vi "Plot_Server_Data.vi"() -> ()   [LabVIEW 2015]
uses:
  Anemometry/Anemometry Sub Vis/Controls/Server_Comms.ctl
  Anemometry/Anemometry Sub Vis/File/Setup_Filetype.ctl
  Anemometry/Anemometry Sub Vis/Globals/Preference_global.vi
panel:
  out "LastUpdated":string="Tue, May 12, 2015 at 11:28"
  in  "Throwback\n(mins)":dbl format="%.1f"
  in  "Precision":i32=2
  in  "Save 3":bool
  out "Plot 3 Chs":string[](array[string])
  in  "Save 2":bool
  out "Plot 2 Chs":string[](array[string])
  in  "Save 1":bool
  out "Plot 1 Chs":string[](array[string])
  in  "Save plot number":T1(ring)
  in  "Selector 1":i32[](listbox)
  in  "Search 1":string="Null" caption="Search:"
  in  "Search 2":string="Null" caption="Search:"
  in  "Search 3":string="Null" caption="Search:"
  out "Plot 3":cluster{"Times":dbl[], "Output array":dbl[]}[](graph)
  in  "Selector 3":i32[](listbox)
  out "Plot 2":cluster{"Times":dbl[], "Output array":dbl[]}[](graph)
  in  "Selector 2":i32[](listbox)
  in  "stop":bool=TRUE
  in  "Mode":T2(ring)=enum."Display data over specified period:"
  out "Plot 1":cluster{"Times":dbl[], "Output array":dbl[]}[](graph)
  in  "History\n(mins)":dbl=20.0 format="%.1f"
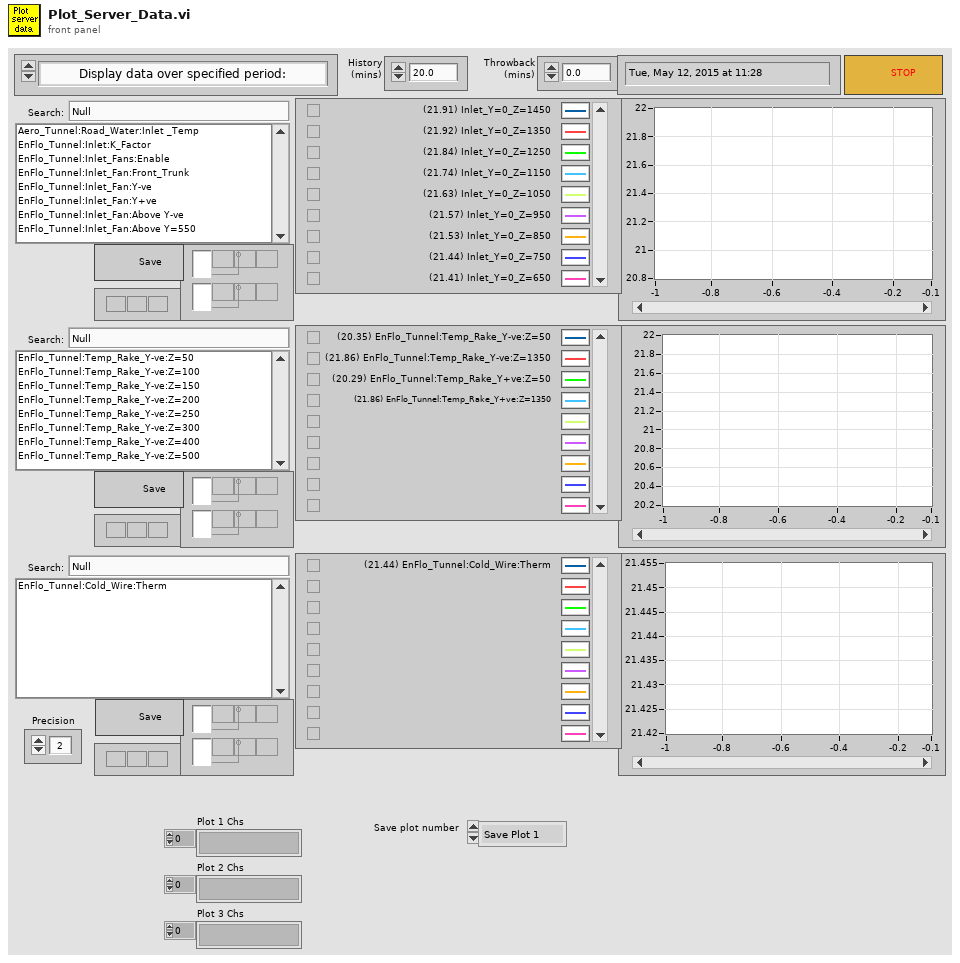
[diagram p1: front panel]
types:
  T1 = enum16{"Save Plot 1", "Save Plot 2", "Save Plot 3"}
  T2 = enum16{"Display full time history", "Display data over specified period:"}
  T3 = typedef "Server_Comms.ctl" = enum16{"Server Link Healthy", "Do Not Link To Server"}
  T4 = typedef "Setup_Filetype.ctl" = enum16{"Measurement Setups", "Calibration Setups", "General", "Results File Plotter Setups", "Speed Calib Tweaks"}
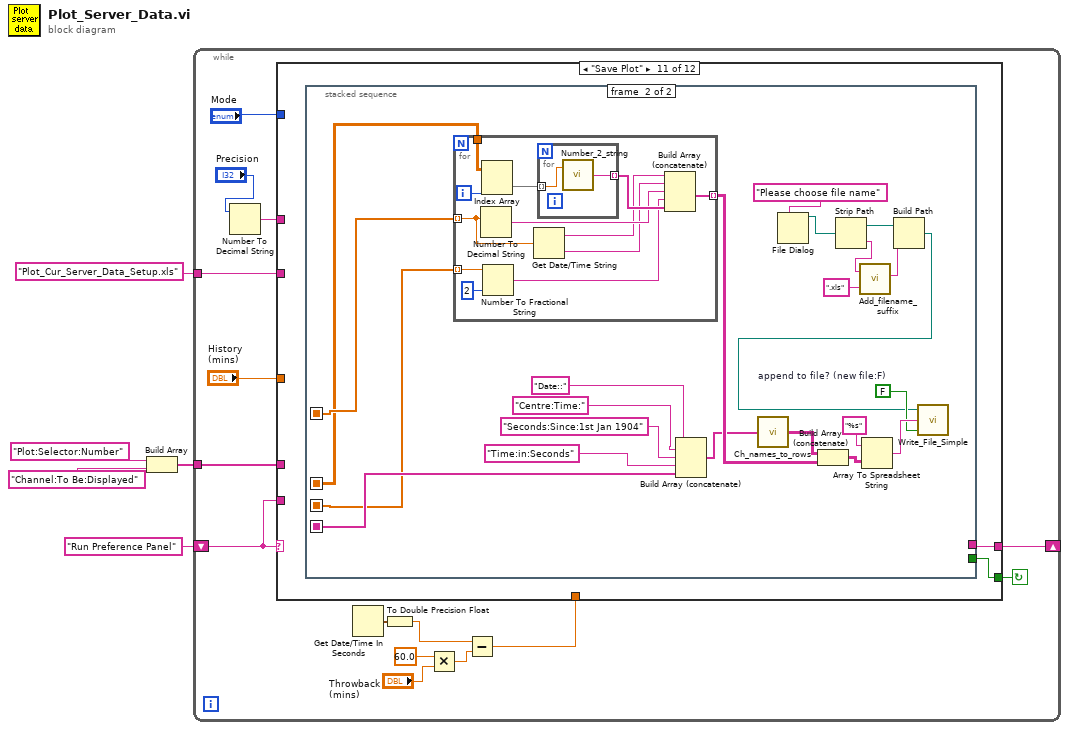
[diagram p0: block diagram]
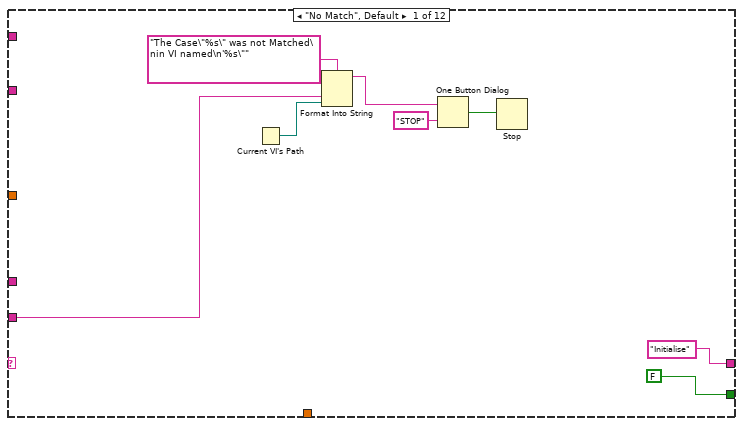
[diagram p2: hidden frame]
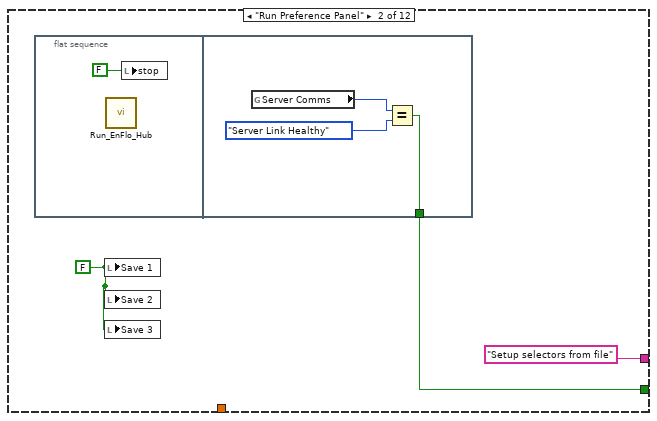
[diagram p3: hidden frame]
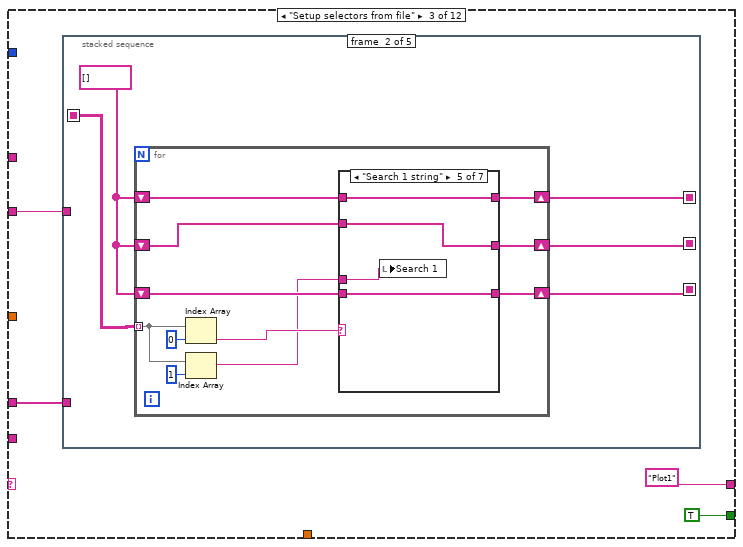
[diagram p4: hidden frame]
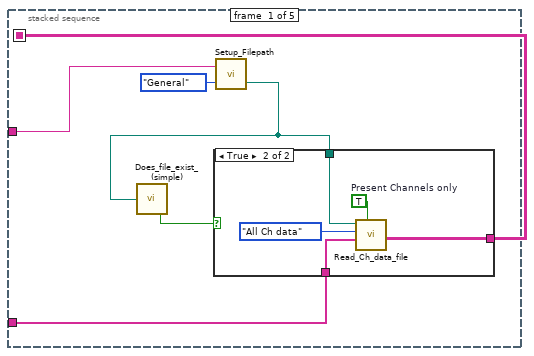
[diagram p5: hidden frame]
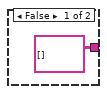
[diagram p6: hidden frame]
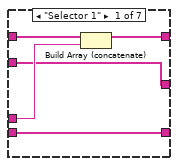
[diagram p7: hidden frame]
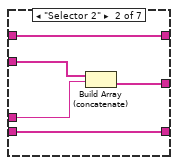
[diagram p8: hidden frame]
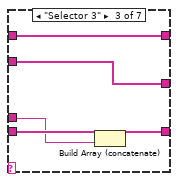
[diagram p9: hidden frame]
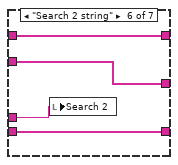
[diagram p11: hidden frame]
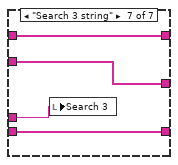
[diagram p12: hidden frame]
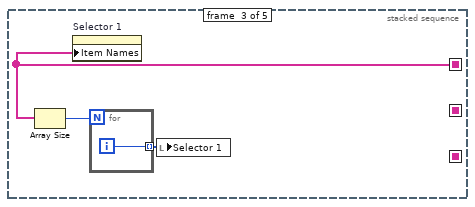
[diagram p13: hidden frame]
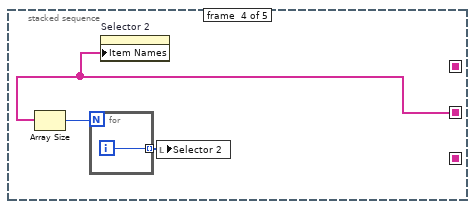
[diagram p14: hidden frame]
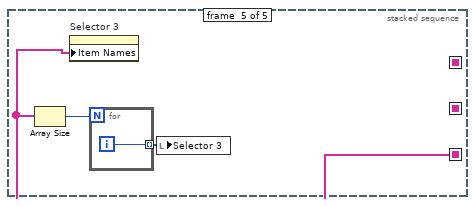
[diagram p15: hidden frame]
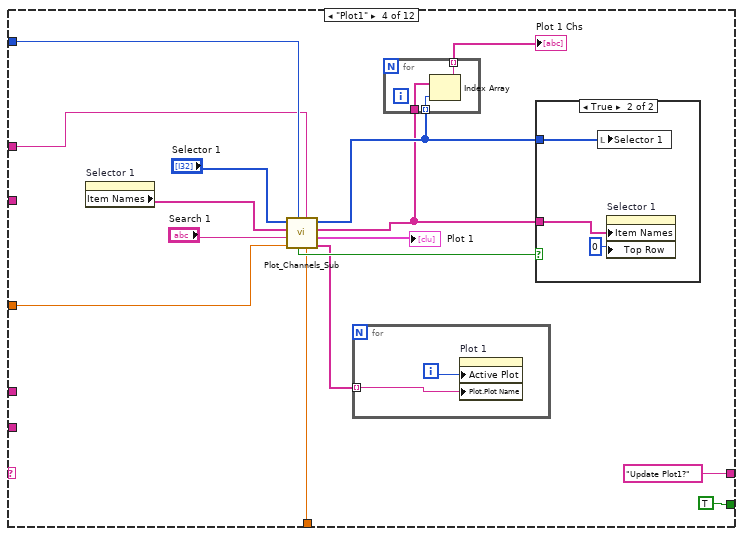
[diagram p16: hidden frame]
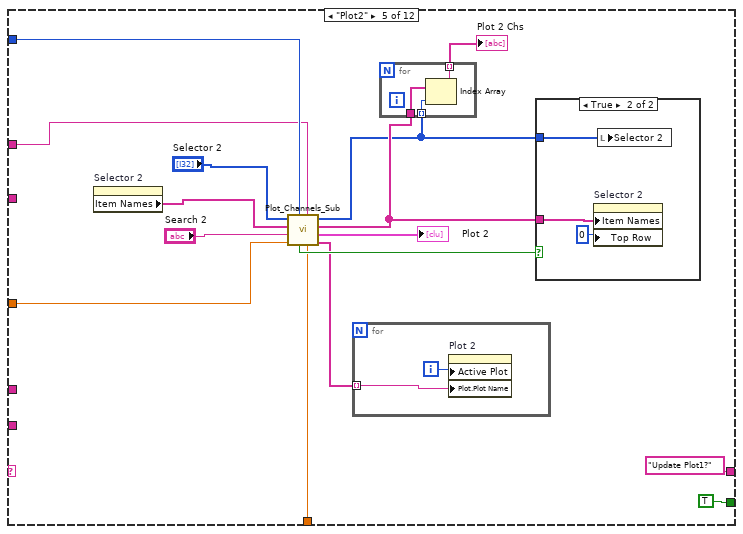
[diagram p18: hidden frame]
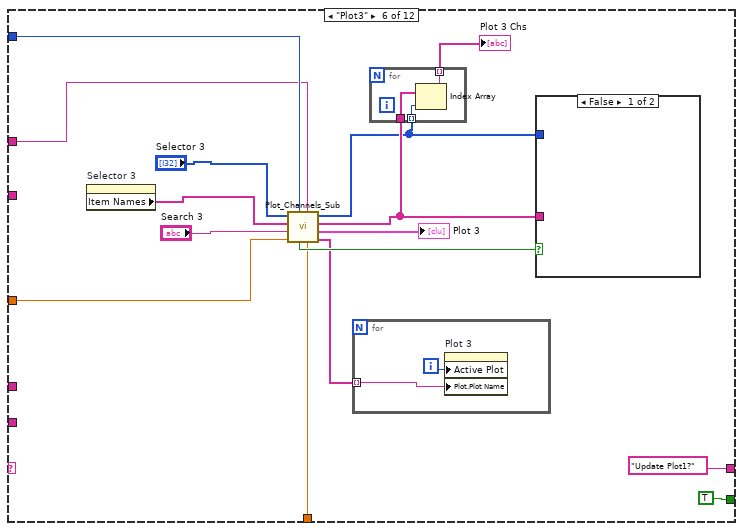
[diagram p20: hidden frame]
diagram:
  n1 = Build Array("Plot:Selector:Number", "Channel:To Be:Displayed") -> (w2:string[])
  n2 = while {
    shift-left: "Run Preference Panel" -> [w18]
    shift-right: [w19] -> _
    tunnel: w2 -> [w15]
    tunnel: "Plot_Cur_Server_Data_Setup.xls" -> [w14]
    stop <- w20 continue-if-true
    n3 = Number To Decimal String(number="Precision") -> (decimal integer string=w12:string)  [unwired: 1 out]
    n4 = Get Date/Time In Seconds() -> (seconds since 1Jan1904=w11:timestamp)
    n5 = To Double Precision Float(number=w11) -> (double precision float=w7:dbl)
    n6 = Multiply(x=60.0, y="Throwback\n(mins)") -> (x*y=w8:dbl)
    n7 = Subtract(x=w7, y=w8) -> (x-y=w6:dbl)
    n8 = case shown="\"Save Plot\"" w18 {
      tunnel: [FALSE w30 TRUE TRUE TRUE TRUE TRUE TRUE TRUE TRUE w305 w370] -> w20
      tunnel: ["Initialise" "Setup selectors from file" "Plot1" "Update Plot1?" "Update Plot1?" "Update Plot1?" w180 w201 w221 w253 w306 "Update Plot1?" ("t")] -> w19
      tunnel: w18 -> [w23 _ _ _ _ _ _ _ _ _ _ _]
      tunnel: "Mode" -> [_ _ _ w117 w144 w167 _ _ _ _ _ _]
      tunnel: "History\n(mins)" -> [_ _ _ w116 w143 w166 _ _ _ _ _ _]
      tunnel: w15 -> [_ _ w36 _ _ _ _ _ _ _ _ w374]
      tunnel: w14 -> [_ _ w37 _ _ _ _ _ _ _ _ w373]
      tunnel: w12 -> [_ _ _ w111 w134 w157 _ _ _ _ _ _]
      tunnel: w6 -> [_ _ _ w110 w133 w156 _ _ _ _ _ _]
      frame "No Match", Default {
        n9 = Current VI's Path() -> (path=w22:path)
        n10 = Format Into String(format string="The Case\"%s\" was not Matched\nin VI named\n'%s\"" ("Format String"), w23, w22) -> (resulting string=w26:string)  [unwired: 2 in, 1 out]
        n11 = One Button Dialog(message=w26, button name ("OK")="STOP") -> (true=w24:bool)
        n12 = Stop(stop? (T)=w24) -> ()
      }
      frame "Run Preference Panel" {
        w29 = FALSE ("Save 1")
        n13 = flat-sequence {
          tunnel: [w33] -> w30
          frame #0 {
            n14 = call "Run_EnFlo_Hub.vi"() -> ()  [unwired: 8 out]
            n15 = local write "stop"(FALSE ("stop")) -> ()
          }
          frame #1 {
            n16 = global read "Preference_global.vi" "Server Comms"() -> (w34:T3)
            n17 = Equal?(x=w34, y=Server_Comms."Server Link Healthy" ("Server Comms")) -> (x = y?=w33:bool)
          }
        }
        n18 = local write "Save 1"(w29) -> ()
        n19 = local write "Save 2"(w29) -> ()
        n20 = local write "Save 3"(w29) -> ()
      }
      frame "Setup selectors from file" {
        n21 = stacked-sequence {
          seq-local: [w43 _ _ _ _] -> [_ w56 _ _ _]
          seq-local: [_ w54 _ _ _] -> [_ _ w100 _ _]
          seq-local: [_ w52 _ _ _] -> [_ _ _ w102 _]
          seq-local: [_ w53 _ _ _] -> [_ _ _ _ w106]
          tunnel: w37 -> [w42 _ _ _ _]
          tunnel: w36 -> [w44 _ _ _ _]
          frame #0 {
            n22 = call "Setup_Filepath.vi"("Setup File Type"=Setup_Filetype."General", "Filename in"=w42) -> ("Filename Out"=w41:path)  [unwired: 1 out]
            n23 = call "Does_file_exist_(simple).vi"("Pathname"=w41) -> ("exists?"=w45:bool)
            n24 = case shown="True" w45 {
              tunnel: w41 -> [_ w51]
              tunnel: w44 -> [_ w50]
              tunnel: [string[][] [] ("Channel Values") w47] -> w43
              frame False {
              }
              frame True {
                w49 = TRUE  # Present Channels only
                n25 = call "Read_Ch_data_file.vi"("Present Channels only"=w49, "Present Channels"=w50, "Output"=enum16{"All Ch data", "The last few rows"}."All Ch data", "Filename"=w51) -> ("Channel Values"=w47:string[][])  [unwired: 1 in, 4 out]
              }
            }
          }
          frame #1 {
            w55 = string[] []
            n26 = for {
              shift-right: [w62] -> w54
              shift-left: w55 -> [w63]
              tunnel: w56 -> [w64] mode=indexing
              shift-right: [w60] -> w52
              shift-left: w55 -> [w61]
              shift-right: [w58] -> w53
              shift-left: w55 -> [w59]
              n27 = Index Array(array=w64, index=0 ("Index")) -> (element=w66:string)
              n28 = Index Array(array=w64, index=1 ("Index")) -> (element=w57:string)
              n29 = case shown="\"Search 1 string\"" w66 {
                tunnel: w63 -> [w72 w77 w78 w84 w88 w92 w96]
                tunnel: [w71 w77 w78 w84 w88 w92 w96] -> w62
                tunnel: w57 -> [w70 w74 w80 _ w86 w90 w94]
                tunnel: w61 -> [w69 w75 w79 w85 w89 w93 w97]
                tunnel: [w69 w73 w79 w85 w89 w93 w97] -> w60
                tunnel: w59 -> [w68 w76 w82 w83 w87 w91 w95]
                tunnel: [w68 w76 w81 w83 w87 w91 w95] -> w58
                frame "Selector 1" {
                  n30 = Build Array (concatenate)(w72, w70) -> (w71:string[])
                }
                frame "Selector 2" {
                  n31 = Build Array (concatenate)(w75, w74) -> (w73:string[])
                }
                frame "Selector 3" {
                  n32 = Build Array (concatenate)(w82, w80) -> (w81:string[])
                }
                frame "No Match", Default {
                }
                frame "Search 1 string" {
                  n33 = local write "Search 1"(w86) -> ()
                }
                frame "Search 2 string" {
                  n34 = local write "Search 2"(w90) -> ()
                }
                frame "Search 3 string" {
                  n35 = local write "Search 3"(w94) -> ()
                }
              }
            }
          }
          frame #2 {
            n36 = Array Size(array=w100) -> (size(s)=w99:i32)
            n37 = property on="Selector 1" class="LstBox (strict)"("Item Names"=w100) -> ()  [unwired: 2 in, 2 out]
            n38 = for {
              N: w99 -> [_]
              tunnel: [w101] -> w98 mode=indexing
              i -> [w101]
            }
            n39 = local write "Selector 1"(w98) -> ()
          }
          frame #3 {
            n40 = Array Size(array=w102) -> (size(s)=w104:i32)
            n41 = for {
              N: w104 -> [_]
              tunnel: [w105] -> w103 mode=indexing
              i -> [w105]
            }
            n42 = property on="Selector 2" class="LstBox (strict)"("Item Names"=w102) -> ()  [unwired: 2 in, 2 out]
            n43 = local write "Selector 2"(w103) -> ()
          }
          frame #4 {
            n44 = Array Size(array=w106) -> (size(s)=w108:i32)
            n45 = property on="Selector 3" class="LstBox (strict)"("Item Names"=w106) -> ()  [unwired: 2 in, 2 out]
            n46 = for {
              N: w108 -> [_]
              tunnel: [w109] -> w107 mode=indexing
              i -> [w109]
            }
            n47 = local write "Selector 3"(w107) -> ()
          }
        }
      }
      frame "Plot1" {
        n48 = property on="Selector 1" class="LstBox (strict)"() -> ("Item Names"=w119:string[])  [unwired: 2 in, 2 out]
        n49 = call "Plot_Channels_Sub.vi"("End Time"=w110, "precision"=w111, "Mode"=w117, "History (min)"=w116, "Search String"="Search 1", "Selector List In"=w119, "Selector array In"="Selector 1") -> ("Plot Legend"=w115:string[], "Plot"=→"Plot 1":cluster{"Times":dbl[], "Output array":dbl[]}[], "Selector List Out"=w113:string[], "Selector array Out"=w114:i32[], "Selector Changed?"=w121:bool)
        n50 = for {
          tunnel: w115 -> [w128] mode=indexing
          i -> [w129]
          n51 = property on="Plot 1" class="XYGraph (strict)"("Active Plot"=w129, "Plot.Plot Name"=w128) -> ()  [unwired: 2 in, 2 out]
        }
        n52 = for {
          tunnel: w114 -> [w127] mode=indexing
          tunnel: w113 -> [w126]
          tunnel: [w125] -> w112 mode=indexing
          n53 = Index Array(array=w126, index=w127) -> (element=w125:string)
        }
        "Plot 1 Chs" <- w112
        n54 = case shown="True" w121 {
          tunnel: w113 -> [_ w132]
          tunnel: w114 -> [_ w131]
          frame False {
          }
          frame True {
            n55 = local write "Selector 1"(w131) -> ()
            n56 = property on="Selector 1" class="LstBox (strict)"("Item Names"=w132, "Top Row"=0) -> ()  [unwired: 2 in, 2 out]
          }
        }
      }
      frame "Plot2" {
        n57 = property on="Selector 2" class="LstBox (strict)"() -> ("Item Names"=w139:string[])  [unwired: 2 in, 2 out]
        n58 = call "Plot_Channels_Sub.vi"("End Time"=w133, "precision"=w134, "Mode"=w144, "History (min)"=w143, "Search String"="Search 2", "Selector List In"=w139, "Selector array In"="Selector 2") -> ("Plot Legend"=w138:string[], "Plot"=→"Plot 2":cluster{"Times":dbl[], "Output array":dbl[]}[], "Selector List Out"=w137:string[], "Selector array Out"=w136:i32[], "Selector Changed?"=w145:bool)
        n59 = for {
          tunnel: w138 -> [w151] mode=indexing
          i -> [w152]
          n60 = property on="Plot 2" class="XYGraph (strict)"("Active Plot"=w152, "Plot.Plot Name"=w151) -> ()  [unwired: 2 in, 2 out]
        }
        n61 = for {
          tunnel: w136 -> [w150] mode=indexing
          tunnel: w137 -> [w149]
          tunnel: [w148] -> w135 mode=indexing
          n62 = Index Array(array=w149, index=w150) -> (element=w148:string)
        }
        "Plot 2 Chs" <- w135
        n63 = case shown="True" w145 {
          tunnel: w137 -> [_ w154]
          tunnel: w136 -> [_ w155]
          frame False {
          }
          frame True {
            n64 = property on="Selector 2" class="LstBox (strict)"("Item Names"=w154, "Top Row"=0) -> ()  [unwired: 2 in, 2 out]
            n65 = local write "Selector 2"(w155) -> ()
          }
        }
      }
      frame "Plot3" {
        n66 = property on="Selector 3" class="LstBox (strict)"() -> ("Item Names"=w162:string[])  [unwired: 2 in, 2 out]
        n67 = call "Plot_Channels_Sub.vi"("End Time"=w156, "precision"=w157, "Mode"=w167, "History (min)"=w166, "Search String"="Search 3", "Selector List In"=w162, "Selector array In"="Selector 3") -> ("Plot Legend"=w161:string[], "Plot"=→"Plot 3":cluster{"Times":dbl[], "Output array":dbl[]}[], "Selector List Out"=w160:string[], "Selector array Out"=w159:i32[], "Selector Changed?"=w168:bool)
        n68 = for {
          tunnel: w161 -> [w174] mode=indexing
          i -> [w175]
          n69 = property on="Plot 3" class="XYGraph (strict)"("Active Plot"=w175, "Plot.Plot Name"=w174) -> ()  [unwired: 2 in, 2 out]
        }
        n70 = for {
          tunnel: w159 -> [w173] mode=indexing
          tunnel: w160 -> [w172]
          tunnel: [w171] -> w158 mode=indexing
          n71 = Index Array(array=w172, index=w173) -> (element=w171:string)
        }
        "Plot 3 Chs" <- w158
        n72 = case shown="False" w168 {
          tunnel: w160 -> [_ w177]
          tunnel: w159 -> [_ w178]
          frame False {
          }
          frame True {
            n73 = local write "Selector 3"(w178) -> ()
            n74 = property on="Selector 3" class="LstBox (strict)"("Item Names"=w177, "Top Row"=0) -> ()  [unwired: 2 in, 2 out]
          }
        }
      }
      frame "Update Plot1?" {
        n75 = while {
          shift-right: [w198] -> w187
          shift-left: _ -> [w195]
          shift-right: [w197] -> w189
          shift-left: _ -> [w196]
          tunnel: [w196] -> w188
          tunnel: [w195] -> w186
          stop <- FALSE continue-if-true
          n76 = local read "Selector 1"() -> (w198:i32[])
          n77 = local read "Search 1"() -> (w197:string)
        }
        n78 = case shown="False" "Save 1" {
          tunnel: ["Update Plot2?" "Save Plot" ("t")] -> w179
          frame False {
          }
          frame True {
            n79 = local write "Save plot number"(T1."Save Plot 1" ("Save plot number")) -> ()
          }
        }
        n80 = Equal?(x=w187, y=w186) -> (x = y?=w184:bool)
        n81 = Equal?(x=w188, y=w189) -> (x = y?=w185:bool)
        n82 = And(x=w184, y=w185) -> (x .and. y?=w183:bool)
        n83 = Select(t=w179, s=w183, f="Plot1") -> (s? t:f=w180:string)
      }
      frame "Update Plot2?" {
        n84 = while {
          shift-right: [w218] -> w207
          shift-left: _ -> [w215]
          shift-right: [w217] -> w209
          shift-left: _ -> [w216]
          tunnel: [w216] -> w208
          tunnel: [w215] -> w206
          stop <- FALSE continue-if-true
          n85 = local read "Selector 2"() -> (w218:i32[])
          n86 = local read "Search 2"() -> (w217:string)
        }
        n87 = case shown="False" "Save 2" {
          tunnel: ["Update Plot3?" "Save Plot" ("t")] -> w199
          frame False {
          }
          frame True {
            n88 = local write "Save plot number"(T1."Save Plot 2" ("Save plot number")) -> ()
          }
        }
        n89 = Equal?(x=w207, y=w206) -> (x = y?=w204:bool)
        n90 = Equal?(x=w208, y=w209) -> (x = y?=w205:bool)
        n91 = And(x=w204, y=w205) -> (x .and. y?=w203:bool)
        n92 = Select(t=w199, s=w203, f="Plot2") -> (s? t:f=w201:string)
      }
      frame "Update Plot3?" {
        n93 = while {
          shift-right: [w238] -> w227
          shift-left: _ -> [w235]
          shift-right: [w237] -> w229
          shift-left: _ -> [w236]
          tunnel: [w236] -> w228
          tunnel: [w235] -> w226
          stop <- FALSE continue-if-true
          n94 = local read "Selector 3"() -> (w238:i32[])
          n95 = local read "Search 3"() -> (w237:string)
        }
        n96 = case shown="False" "Save 3" {
          tunnel: ["What to do next?" "Save Plot" ("t")] -> w219
          frame False {
          }
          frame True {
            n97 = local write "Save plot number"(T1."Save Plot 3" ("Save plot number")) -> ()
          }
        }
        n98 = Equal?(x=w227, y=w226) -> (x = y?=w224:bool)
        n99 = Equal?(x=w228, y=w229) -> (x = y?=w225:bool)
        n100 = And(x=w224, y=w225) -> (x .and. y?=w223:bool)
        n101 = Select(t=w219, s=w223, f="Plot3") -> (s? t:f=w221:string)
      }
      frame "What to do next?" {
        n102 = Wait (ms)(milliseconds to wait=u32 300) -> ()  [unwired: 1 out]
        n103 = while {
          shift-right: [w269] -> _
          shift-left: _ -> [w268]
          shift-right: [w267] -> _
          shift-left: _ -> [w266]
          shift-right: [w259] -> _
          shift-left: _ -> [w258]
          tunnel: [w261] -> w252
          shift-right: [w255] -> w241
          shift-left: _ -> [w256]
          stop <- FALSE continue-if-true
          n104 = local read "History\n(mins)"() -> (w269:dbl)
          n105 = local read "Mode"() -> (w267:T2)
          n106 = Equal?(x=w269, y=w268) -> (x = y?=w265:bool)
          n107 = Equal?(x=w266, y=w267) -> (x = y?=w264:bool)
          n108 = And(x=w265, y=w264) -> (x .and. y?=w263:bool)
          n109 = Select(t=w258, s=w263, f=0) -> (s? t:f=w260:i32)
          n110 = case shown="2" w260 {
            tunnel: ["Plot1" "Plot2" "Plot3" "Update Plot1?" "Update Plot1?" "Update Plot1?" "Update Plot1?"] -> w261
            tunnel: w260 -> [w272 w276 w280 w286 w292 w298 _]
            tunnel: [w271 w275 w279 w285 w291 w297 0] -> w259
            tunnel: w256 -> [w270 w274 w278 w283 w289 w294 w301]
            tunnel: [w270 w274 w278 w282 w288 w295 w300] -> w255
            frame 0, Default {
              n111 = Increment(x=w272) -> (x+1=w271:i32)
            }
            frame 1 {
              n112 = Increment(x=w276) -> (x+1=w275:i32)
            }
            frame 2 {
              n113 = Increment(x=w280) -> (x+1=w279:i32)
            }
            frame 3 {
              n114 = Add(x=w283, y=1) -> (x+y=w282:i32)
              n115 = Increment(x=w286) -> (x+1=w285:i32)
            }
            frame 4 {
              n116 = Add(x=w289, y=1) -> (x+y=w288:i32)
              n117 = Increment(x=w292) -> (x+1=w291:i32)
            }
            frame 5 {
              n118 = Add(x=w294, y=1) -> (x+y=w295:i32)
              n119 = Increment(x=w298) -> (x+1=w297:i32)
            }
            frame 6 {
              n120 = Add(x=w301, y=1) -> (x+y=w300:i32)
            }
          }
        }
        n121 = Get Date/Time String(date format (0)=enum16{"short", "long", "abbreviated"}."abbreviated") -> (date string=w248:string, time string=w249:string)  [unwired: 2 out]
        n122 = Concatenate Strings(w248, " at " ("Substring"), w249) -> (→"LastUpdated":string)
        n123 = Quotient & Remainder(x=w241, y=500) -> (x-y*floor(x/y)=w245:i32)  [unwired: 1 out]
        n124 = Equal To 0?(x=w245) -> (x = 0?=w243:bool)
        n125 = Or(x="stop", y=w243) -> (x .or. y?=w242:bool)
        n126 = Select(t="Save Channel Names", s=w242, f=w252) -> (s? t:f=w253:string)
      }
      frame "Save Plot" {
        n127 = stacked-sequence {
          seq-local: [w317 _] -> [_ w345]
          seq-local: [w312 _] -> [_ w347]
          seq-local: [w316 _] -> [_ w346]
          seq-local: [w307 _] -> [_ w335]
          tunnel: ["What to do next?" _] -> w306
          tunnel: [TRUE _] -> w305
          frame #0 {
            n128 = case shown="\"Save Plot 1\"" "Save plot number" {
              tunnel: [w325 w328 w331] -> w322
              tunnel: [w324 w327 w330] -> w317
              frame "Save Plot 1" {
                n129 = local read "Plot 1 Chs"() -> (w324:string[])
                n130 = local write "Save 1"(FALSE ("Save 1")) -> ()
                n131 = local read "Plot 1"() -> (w325:cluster{"Times":dbl[], "Output array":dbl[]}[])
              }
              frame "Save Plot 2" {
                n132 = local read "Plot 2 Chs"() -> (w327:string[])
                n133 = local write "Save 2"(FALSE ("Save 1")) -> ()
                n134 = local read "Plot 2"() -> (w328:cluster{"Times":dbl[], "Output array":dbl[]}[])
              }
              frame "Save Plot 3" {
                n135 = local read "Plot 3 Chs"() -> (w330:string[])
                n136 = local write "Save 3"(FALSE ("Save 1")) -> ()
                n137 = local read "Plot 3"() -> (w331:cluster{"Times":dbl[], "Output array":dbl[]}[])
              }
            }
            n138 = Index Array(array=w322, index=0) -> (element=w320:cluster{"Times":dbl[], "Output array":dbl[]})
            n139 = Unbundle(w320) -> ("Times"=w311:dbl[])  [unwired: 1 out]
            n140 = Get Date/Time In Seconds() -> (seconds since 1Jan1904=w314:timestamp)
            n141 = for {
              tunnel: w322 -> [w333] mode=indexing
              tunnel: [w332] -> w316 mode=indexing
              n142 = Unbundle(w333) -> ("Output array"=w332:dbl[])  [unwired: 1 out]
            }
            n143 = To Double Precision Float(number=w314) -> (double precision float=w313:dbl)
            n144 = Multiply(x=w311, y=60.0) -> (x*y=w309:dbl[])
            n145 = Add(x=w313, y=w309) -> (x+y=w312:dbl[])
            n146 = Index Array(array=w309) -> (element=w308:dbl)  [unwired: 1 in]
            n147 = Subtract(x=w309, y=w308) -> (x-y=w307:dbl[])
          }
          frame #1 {
            w340 = FALSE  # append to file? (new file:F)
            n148 = for {
              tunnel: w346 -> [w367]
              tunnel: w347 -> [w361] mode=indexing
              tunnel: [w363] -> w339 mode=indexing
              tunnel: w335 -> [w357] mode=indexing
              i -> [w366]
              n149 = Number To Decimal String(number=w361) -> (decimal integer string=w362:string)  [unwired: 1 out]
              n150 = Index Array(array=w367, index (col)=w366) -> (element=w365:dbl[])  [unwired: 1 in]
              n151 = Number To Fractional String(number=w357, precision (6)=i16 2) -> (F-format string=w356:string)  [unwired: 2 in]
              n152 = Get Date/Time String(seconds (now)=w361) -> (date string=w360:string, time string=w359:string)  [unwired: 2 out]
              n153 = for {
                tunnel: w365 -> [w369] mode=indexing
                tunnel: [w368] -> w364 mode=indexing
                n154 = call "Number_2_string.vi"("number"=w369) -> ("String"=w368:string)  [unwired: 1 in]
              }
              n155 = Build Array (concatenate)(w360, w359, w362, w356, w364) -> (w363:string[])
            }
            n156 = Build Array (concatenate)("Date::", "Centre:Time:", "Seconds:Since:1st Jan 1904", "Time:in:Seconds", w345) -> (w338:string[])
            n157 = call "Ch_names_to_rows.vi"("Channel Names"=w338) -> ("3 Row names"=w344:string[][])
            n158 = File Dialog(7:"Please choose file name" ("prompt")) -> (3:w352:path)  [unwired: 1 in, 8 out]
            n159 = Build Array (concatenate)(w344, w339) -> (w342:string[][])
            n160 = Strip Path(path=w352) -> (stripped path=w349:path, name=w351:string)
            n161 = call "Add_filename_suffix.vi"("Filename"=w351, "Suffix to add"=".xls") -> ("Filename out"=w348:string)  [unwired: 3 out]
            n162 = Array To Spreadsheet String(array=w342, 3:"%s" ("format string")) -> (spreadsheet string=w341:string)  [unwired: 1 out]
            n163 = Build Path(base path=w349, name or relative path=w348) -> (appended path=w337:path)
            n164 = call "Write_File_Simple.vi"("append to file? (new file:F)"=w340, "character string"=w341, "file path"=w337) -> ()  [unwired: 2 out]
          }
        }
      }
      frame "Save Channel Names" {
        n165 = stacked-sequence {
          seq-local: [w376 _ _] -> [_ w400 _]
          seq-local: [_ w399 _] -> [_ _ w413]
          tunnel: w374 -> [_ _ w414]
          tunnel: w373 -> [_ _ w411]
          frame #0 {
            n166 = for {
              N: 3 -> [_]
              shift-right: [w380] -> w376
              shift-left: string[][] [] -> [w382]
              i -> [w387]
              n167 = Increment(x=w387) -> (x+1=w384:i32)
              n168 = case shown="1, Default" w384 {
                tunnel: [w394 w395 w397] -> w386
                tunnel: [w393 w396 w398] -> w378
                frame 1, Default {
                  n169 = local read "Selector 1"() -> (w394:i32[])
                  n170 = property on="Selector 1" class="LstBox (strict)"() -> ("Item Names"=w393:string[])  [unwired: 2 in, 2 out]
                }
                frame 2 {
                  n171 = property on="Selector 2" class="LstBox (strict)"() -> ("Item Names"=w396:string[])  [unwired: 2 in, 2 out]
                  n172 = local read "Selector 2"() -> (w395:i32[])
                }
                frame 3 {
                  n173 = local read "Selector 3"() -> (w397:i32[])
                  n174 = property on="Selector 3" class="LstBox (strict)"() -> ("Item Names"=w398:string[])  [unwired: 2 in, 2 out]
                }
              }
              n175 = Format Into String(format string="%d" ("Format String"), initial string="Selector ", w384) -> (resulting string=w381:string)  [unwired: 1 in, 1 out]
              n176 = for {
                tunnel: w386 -> [w392] mode=indexing
                tunnel: w381 -> [w391]
                tunnel: [w389] -> w379 mode=indexing
                tunnel: w378 -> [w388]
                n177 = Index Array(array=w388, index=w392) -> (element=w390:string)
                n178 = Build Array(w391, w390) -> (w389:string[])
              }
              n179 = Build Array (concatenate)(w382, w379) -> (w380:string[][])
            }
          }
          frame #1 {
            n180 = local read "Search 1"() -> (w401:string)
            n181 = local read "Search 2"() -> (w402:string)
            n182 = local read "Search 3"() -> (w403:string)
            n183 = Build Array("Search 1 string" ("element"), w401) -> (w407:string[])
            n184 = Build Array("Search 3 string" ("element"), w403) -> (w409:string[])
            n185 = Build Array("Search 2 string" ("element"), w402) -> (w408:string[])
            n186 = Build Array (concatenate)(w400, w407, w408, w409) -> (w399:string[][])
          }
          frame #2 {
            n187 = call "Setup_Filepath.vi"("Setup File Type"=Setup_Filetype."General", "Filename in"=w411) -> ("Filename Out"=w410:path)  [unwired: 1 out]
            n188 = Array Size(array=w413) -> (size(s)=w417:i32[])
            n189 = Index Array(array=w417, index=1 ("Index")) -> (element=w416:i32)
            n190 = Not Equal To 0?(x=w416) -> (x != 0?=w415:bool)
            n191 = case shown="True" w415 {
              tunnel: w410 -> [w419 w424]
              tunnel: w413 -> [_ w425]
              tunnel: w414 -> [_ w426]
              frame False {
                n192 = Delete(path (use dialog)=w419) -> ()  [unwired: 1 in, 6 out]
              }
              frame True {
                w420 = FALSE  # append to file? (new file:F)
                n193 = call "Ch_names_to_rows.vi"("Channel Names"=w426) -> ("3 Row names"=w427:string[][])
                n194 = Build Array (concatenate)(w427, w425) -> (w422:string[][])
                n195 = Array To Spreadsheet String(array=w422, 3:"%s" ("format string")) -> (spreadsheet string=w421:string)  [unwired: 1 out]
                n196 = call "Write_File_Simple.vi"("append to file? (new file:F)"=w420, "character string"=w421, "file path"=w424) -> ()  [unwired: 2 out]
              }
            }
          }
        }
        n197 = local read "stop"() -> (w371:bool)
        n198 = Not(x=w371) -> (.not. x?=w370:bool)
      }
    }
  }
